vi "Pause_Acquisition.vi"() -> (0 "Paused":bool)   [LabVIEW 2010]
uses:
  Globals/Trav_pos_global.vi
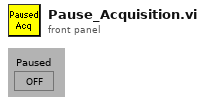
[diagram p1: front panel]
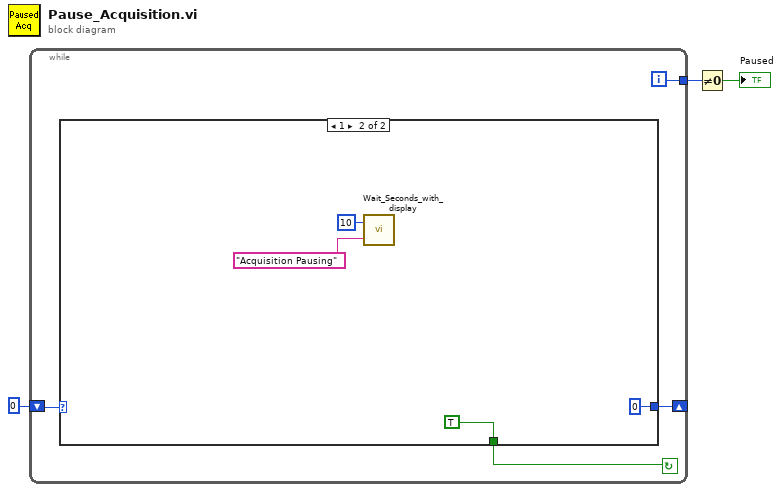
[diagram p0: block diagram]
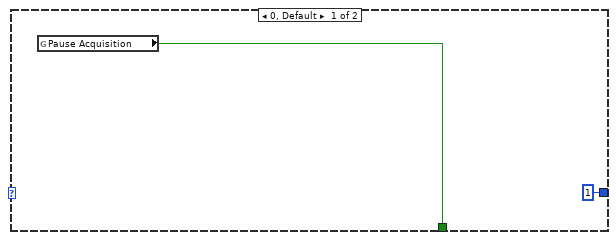
[diagram p2: hidden frame]
diagram:
  n1 = while {
    tunnel: [w4] -> w2
    shift-left: 0 -> [w6]
    shift-right: [w5] -> _
    i -> [w4]
    stop <- w7 continue-if-true
    n2 = case shown="1" w6 {
      tunnel: [w9 TRUE ("Pause Acquisition")] -> w7
      tunnel: [1 0] -> w5
      frame 0, Default {
        n3 = global read "Trav_pos_global.vi" "Pause Acquisition"() -> (w9:bool)
      }
      frame 1 {
        n4 = call "Wait_Seconds_with_display.vi"("Message"="Acquisition Pausing", "Seconds to wait"=u32 10) -> ()  [unwired: 2 out]
      }
    }
  }
  n5 = Not Equal To 0?(x=w2) -> (x != 0?=→"Paused":bool)
